vi "bh3_set_extended_data_packet_transmit_state.vi"(7 "enable?":bool, 8 "error in (no error)":errorcluster, 11 "bt connection ID in":refnum<k31>) -> (0 "error out":errorcluster, 3 "bt connection ID out":refnum<k31>)   [LabVIEW 2013]
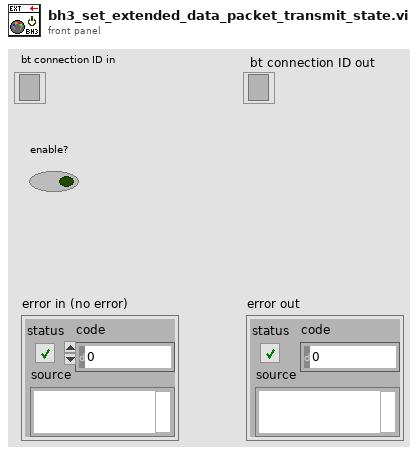
[diagram p1: front panel]
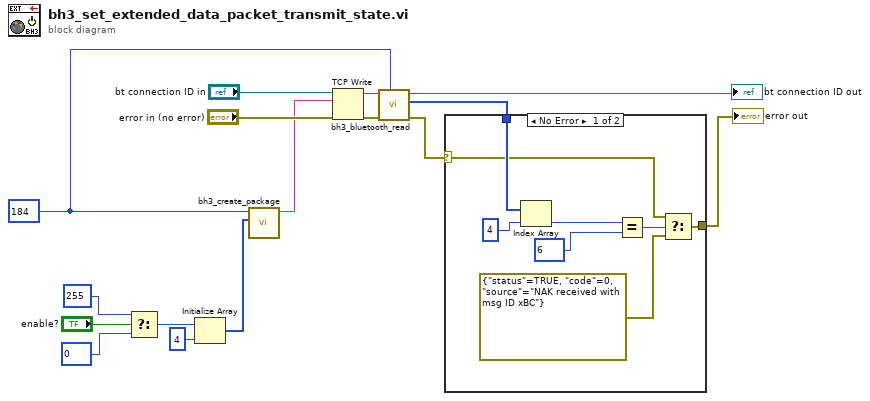
[diagram p0: block diagram]
diagram:
  w4 = u8 184 ("msg_ID")
  n1 = Select(t=u8 255 ("msg_ID"), s="enable?", f=u8 0 ("msg_ID")) -> (s? t:f=w3:u8)
  n2 = Initialize Array(w3, 4 ("dimension size")) -> (w2:u8[])
  n3 = call "bh3_create_package.vi"("Payload"=w2, "msg_ID"=w4) -> ("package string"=w14:string)  [unwired: 8 in, 1 out]
  n4 = TCP Write(connection ID="bt connection ID in", data in=w14, error in (no error)="error in (no error)") -> (connection ID out=w8:refnum<k31>, error out=w10:errorcluster)  [unwired: 1 in, 1 out]
  n5 = call "bh3_bluetooth_read.vi"("command_expected(x00)"=w4, "error in (no error)"=w10, "bt connection ID in"=w8) -> ("error out"=w5:errorcluster, "response byte array"=w7:u8[], "bt connection ID out"=→"bt connection ID out":refnum<k31>)  [unwired: 6 in]
  n6 = case shown="No Error" w5 {
    selector: w5 -> [w17 w25]
    tunnel: w7 -> [w24 _]
    tunnel: [w19 w25] -> w6
    frame No Error {
      n7 = Index Array(array=w24, index=4) -> (element=w22:u8)
      n8 = Equal?(x=w22, y=u8 6 ("msg_ID")) -> (x = y?=w20:bool)
      n9 = Select(t=w17, s=w20, f=errorcluster {"status"=TRUE, "code"=0, "source"="NAK received with msg ID xBC"} ("s? t:f")) -> (s? t:f=w19:errorcluster)
    }
    frame Error {
    }
  }
  "error out" <- w6
